vi "POLARIS Camera.vi"() -> ()   [LabVIEW 2009]
uses:
  XDisplay/POLARIS IMAQ Display.xctl
  Analyze Classes/Analyze Timer/Analyze Timer.lvclass
  XDisplay/Properties/ImageSource.ctl
  IMAQdx Cam/IMAQdx Cam.lvclass
  Utility/POLARIS Vision utility.lvlib
panel:
  in  "stop2":bool
  in  "Energy [J]":dbl
  out "error sett.":errorcluster
  in  "Config Dir":path=path "D:/Test XDisplay images"
  in  "Prefix":string
  in  "WorkDir":path=path "D:/Test XDisplay images"
  out "XDisplay":cluster{"Image":T1}(xcontrol)
  in  "stop":bool
  in  "Camera Name":string="JustageCam"
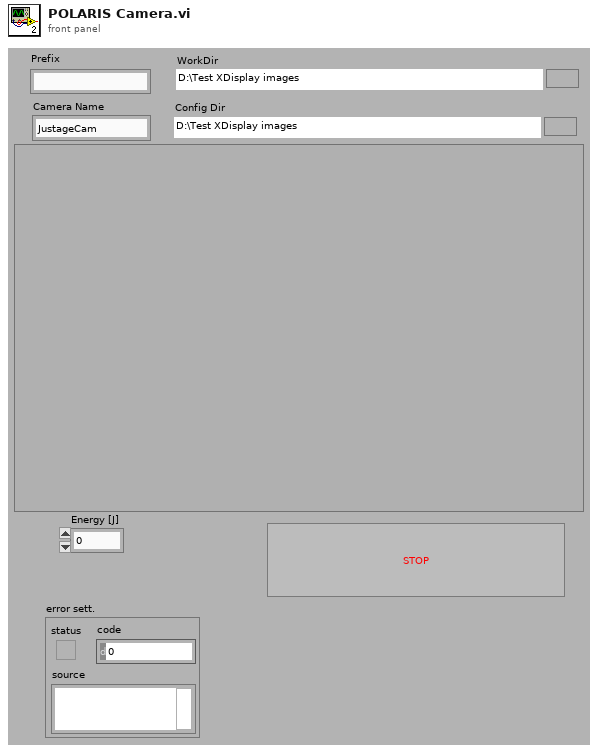
[diagram p1: front panel]
types:
  T1 = typedef "IMAQ Image.ctl" = refnum<image>
  T2 = typedef "POLARIS IMAQ Display.xctl/ImageSource.ctl" = enum16{"Camera", "File"}
  T3 = typedef "Image Type" = u32
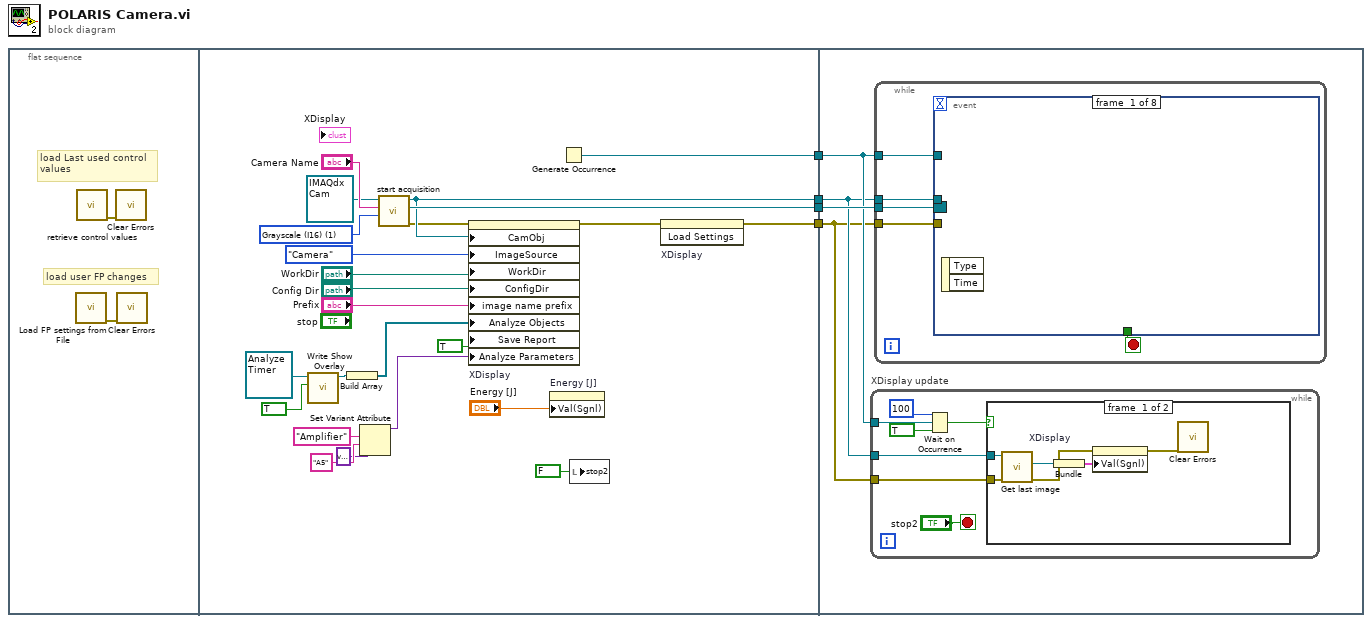
[diagram p0: block diagram]
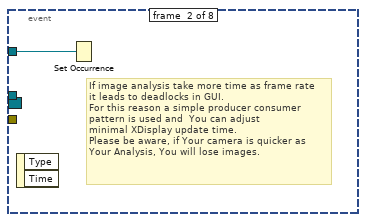
[diagram p3: hidden frame]
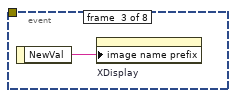
[diagram p4: hidden frame]
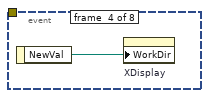
[diagram p5: hidden frame]
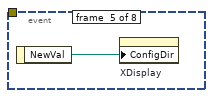
[diagram p6: hidden frame]
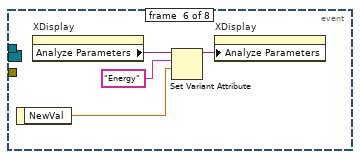
[diagram p7: hidden frame]
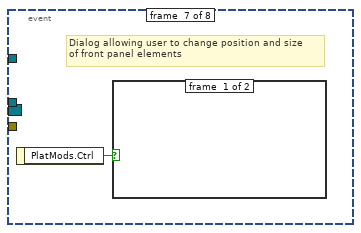
[diagram p8: hidden frame]
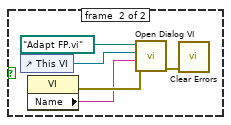
[diagram p9: hidden frame]
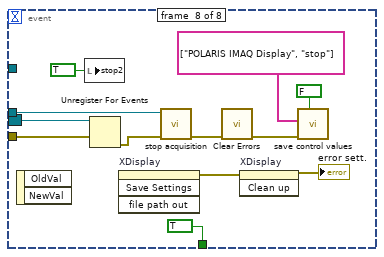
[diagram p10: hidden frame]
diagram:
  n1 = flat-sequence {
    tunnel: [w29] -> w4
    tunnel: [w25] -> w3
    tunnel: [w16] -> w2
    tunnel: [w19] -> w1
    tunnel: w4 -> [w34]
    tunnel: w3 -> [w32]
    tunnel: w2 -> [w31]
    tunnel: w1 -> [w33]
    frame #0 {
      # "load user FP changes"
      # "load Last used control\nvalues"
      n2 = call "Load FP settings from File.vi"() -> ("error out"=w5:errorcluster)  [unwired: 11 in]
      n3 = call "retrieve control values.vi"() -> ("error out"=w6:errorcluster)  [unwired: 10 in, 1 out]
      n4 = call <vilib>:"Clear Errors.vi"("error in (no error)"=w6) -> ()  [unwired: 6 in, 1 out]
      n5 = call <vilib>:"Clear Errors.vi"("error in (no error)"=w5) -> ()  [unwired: 6 in, 1 out]
    }
    frame #1 {
      w23 = T3 1 items=["Grayscale (U8)", "Grayscale (I16)", "Grayscale (SGL)", "Complex (CSG)", "RGB (U32)", "HSL (U32)", "RGB (U64)", "Grayscale (U16)"] ("Image Type")
      n6 = call-dynamic "Write Show Overlay.vi"("Overlay?"=TRUE, "Analyze BaseClass in"=refnum<class "Analyze Timer.lvclass"> refnum ("Analyze Timer.lvclass")) -> ("Analyze BaseClass out"=w12:refnum<class "Analyze Timer.lvclass">)  [unwired: 8 in, 1 out]
      n7 = Build Array(w12) -> (w14:refnum<class "Analyze Timer.lvclass">[])
      n8 = Set Variant Attribute(Variant=variant ("variant"), name="Amplifier", value="A5" ("name")) -> (Variant out=w10:variant)  [unwired: 1 in, 2 out]
      n9 = call-dynamic "start acquisition.vi"("Image Type"=w23, "Camera Name"="Camera Name", "IMAQdx Cam in"=refnum<class "IMAQdx Cam.lvclass"> refnum ("IMAQdx Cam.lvclass")) -> ("error out"=w24:errorcluster, "Event Registration Refnum"=w29:refnum<event-registration>, "IMAQdx Cam out"=w25:refnum<class "IMAQdx Cam.lvclass">)  [unwired: 6 in]
      n10 = property on="XDisplay" class="POLARIS IMAQ Display (strict)"(error in=w24, "CamObj"=w25, "ImageSource"=ImageSource."Camera", "WorkDir"="WorkDir", "ConfigDir"="Config Dir", "image name prefix"="Prefix", "Analyze Objects"=w14, "Save Report"=TRUE, "Analyze Parameters"=w10) -> (error out=w17:errorcluster)  [unwired: 1 in, 1 out]
      n11 = property on="Energy [J]" class="DigNum (strict)"("Val(Sgnl)"="Energy [J]") -> ()  [unwired: 2 in, 2 out]
      n12 = Generate Occurrence() -> (w19:refnum<k4>)
      n13 = local write "stop2"(FALSE ("stop2")) -> ()
      n14 = invoke on="XDisplay" class="POLARIS IMAQ Display (strict)" method="Load Settings"(error in=w17) -> (error out=w16:errorcluster)  [unwired: 2 in, 2 out]
    }
    frame #2 {
      n15 = while "XDisplay update" {
        tunnel: w33 -> [w41]
        tunnel: w32 -> [w38]
        tunnel: w31 -> [w37]
        stop <- "stop2" stop-if-true
        n16 = Wait on Occurrence(1:TRUE ("ignore previous (T)"), 2:w41, 3:100 ("ms timeout (-1)")) -> (0:w39:bool)
        n17 = case shown="False" w39 {
          tunnel: w38 -> [w44 _]
          tunnel: w37 -> [w43 _]
          frame #0 {
            n18 = call-dynamic "Get last image.vi"("error in (no error)"=w43, "IMAQdx Cam in"=w44) -> ("error out"=w46:errorcluster, "Image Out"=w45:T1)  [unwired: 7 in, 1 out]
            n19 = Bundle("Image Out"=w45) -> (w47:cluster{"Image Out":T1})  [unwired: 1 in]
            n20 = property on="XDisplay" class="POLARIS IMAQ Display (strict)"(error in=w46, "Val(Sgnl)"=w47) -> (error out=w42:errorcluster)  [unwired: 1 in, 1 out]
            n21 = call <vilib>:"Clear Errors.vi"("error in (no error)"=w42) -> ()  [unwired: 6 in, 1 out]
          }
          frame #1 {
          }
        }
      }
      n22 = while {
        tunnel: w32 -> [w51]
        tunnel: w34 -> [w50]
        tunnel: w31 -> [w49]
        tunnel: w33 -> [w48]
        stop <- w52 stop-if-true
        n23 = event shown="[5] \"Energy [J]\": Value Change" {
          selector: w50 -> [_ _ _ _ _ _ _ w75]
          dyn-events: _ -> [_ _ _ _ _ _ _ _]
          timeout: _ -> [_ _ _ _ _ _ _ _]
          tunnel: [_ _ _ _ _ _ _ TRUE] -> w52
          tunnel: w51 -> [_ _ _ _ _ _ _ w76]
          tunnel: w49 -> [_ _ _ _ _ _ _ w74]
          tunnel: w48 -> [_ w53 _ _ _ _ _ _]
          event #0 {
            n24 = event-data() -> ()  [unwired: 1 in, 2 out]
          }
          event #1 {
            # "If image analysis take more time as frame rate\nit leads to deadlocks in GUI.\nFor this reason a simple producer consumer \npattern is used and  You can adjust \nminimal XDisplay update time.\nPlease be aware, if Your camera is quicker as\nYour Analysis, You will lose images."
            n25 = event-data() -> ()  [unwired: 1 in, 2 out]
            n26 = Set Occurrence(w53) -> ()
          }
          event #2 {
            n27 = event-data() -> ("NewVal"=w54:string)  [unwired: 1 in]
            n28 = property on="XDisplay" class="POLARIS IMAQ Display (strict)"("image name prefix"=w54) -> ()  [unwired: 2 in, 2 out]
          }
          event #3 {
            n29 = event-data() -> ("NewVal"=w55:path)  [unwired: 1 in]
            n30 = property on="XDisplay" class="POLARIS IMAQ Display (strict)"("WorkDir"=w55) -> ()  [unwired: 2 in, 2 out]
          }
          event #4 {
            n31 = event-data() -> ("NewVal"=w56:path)  [unwired: 1 in]
            n32 = property on="XDisplay" class="POLARIS IMAQ Display (strict)"("ConfigDir"=w56) -> ()  [unwired: 2 in, 2 out]
          }
          event #5 {
            n33 = event-data() -> ("NewVal"=w57:dbl)  [unwired: 1 in]
            n34 = property on="XDisplay" class="POLARIS IMAQ Display (strict)"() -> ("Analyze Parameters"=w60:variant)  [unwired: 2 in, 2 out]
            n35 = Set Variant Attribute(Variant=w60, name="Energy", value=w57) -> (Variant out=w58:variant)  [unwired: 1 in, 2 out]
            n36 = property on="XDisplay" class="POLARIS IMAQ Display (strict)"("Analyze Parameters"=w58) -> ()  [unwired: 2 in, 2 out]
          }
          event #6 {
            # "Dialog allowing user to change position and size\nof front panel elements"
            n37 = event-data() -> ("PlatMods.Ctrl"=w61:bool)  [unwired: 1 in]
            n38 = case shown="True" w61 {
              frame #0 {
              }
              frame #1 {
                n39 = control-ref of="This VI"() -> (w65:refnum<vi>)
                n40 = property class="VI"() -> (error out=w64:errorcluster, "Name"=w63:string)  [unwired: 2 in, 1 out]
                n41 = call "Open Dialog VI.vi"("error in"=w64, "Windows title"=w63, "ref for signalling"=w65, "vi path"=path "Adapt FP.vi") -> ("error out"=w62:errorcluster)  [unwired: 7 in]
                n42 = call <vilib>:"Clear Errors.vi"("error in (no error)"=w62) -> ()  [unwired: 6 in, 1 out]
              }
            }
          }
          event #7 {
            n43 = event-data() -> ()  [unwired: 1 in, 2 out]
            n44 = local write "stop2"(TRUE ("stop2")) -> ()
            n45 = Unregister For Events(event registration refnum=w75, error in=w74) -> (error out=w77:errorcluster)
            n46 = invoke on="XDisplay" class="POLARIS IMAQ Display (strict)" method="Save Settings"() -> (error out=w68:errorcluster)  [unwired: 4 in, 3 out]
            n47 = call-dynamic "stop acquisition.vi"("error in (no error)"=w77, "IMAQdx Cam in"=w76) -> ("error out"=w73:errorcluster)  [unwired: 8 in, 1 out]
            n48 = call <vilib>:"Clear Errors.vi"("error in (no error)"=w73) -> ("error out"=w72:errorcluster)  [unwired: 6 in]
            n49 = invoke on="XDisplay" class="POLARIS IMAQ Display (strict)" method="Clean up"(error in=w68) -> (error out=→"error sett.":errorcluster)  [unwired: 2 in, 2 out]
            n50 = call "save control values.vi"("Append timestamp (true)"=FALSE, "error in"=w72, "Dont save"=string[] ["POLARIS IMAQ Display", "stop"]) -> ()  [unwired: 5 in, 2 out]
          }
        }
      }
    }
  }
